vi "Set View.vi"(8 "error in":errorcluster, 10 "CellView":refnum<class "Cell View.lvclass">, 11 "Cell in":refnum<class "Cell.lvclass">) -> (0 "error out":errorcluster, 3 "Cell out":refnum<class "Cell.lvclass">)   [LabVIEW 2023, in "SourceGrid.lvlib" / "Cell.lvclass"]
uses:
  Cell.lvclass
  Views/Cell View/Cell View.lvclass
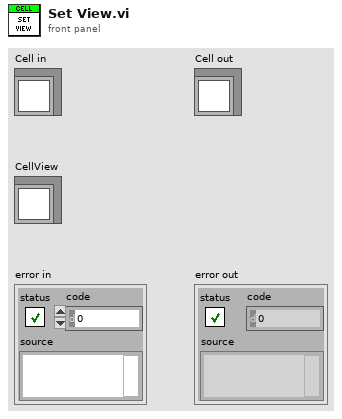
[diagram p1: front panel]
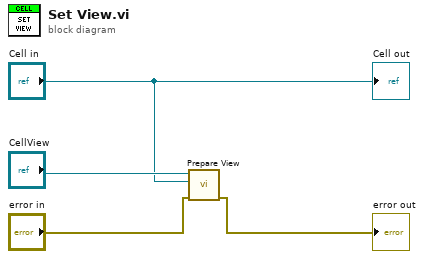
[diagram p0: block diagram]
diagram:
  n1 = call-dynamic "Prepare View.vi"("error in"="error in", "Cell"="Cell in", "Cell View in"="CellView") -> ("error out"=→"error out":errorcluster)  [unwired: 7 in, 1 out]
  "Cell out" <- "Cell in"
